vi "Write connect timeout ms.vi"(8 "error in (no error)":errorcluster, 10 "connect timeout ms":i32, 11 "TCP Master in":refnum<class "TCP Master.lvclass">) -> (0 "error out":errorcluster, 3 "TCP Master out":refnum<class "TCP Master.lvclass">)   [LabVIEW 2013, in "Modbus Library - Advance.lvlib" / "TCP Master.lvclass"]
uses:
  TCP Master.lvclass
  TCP Master.lvclass/TCP Master.ctl
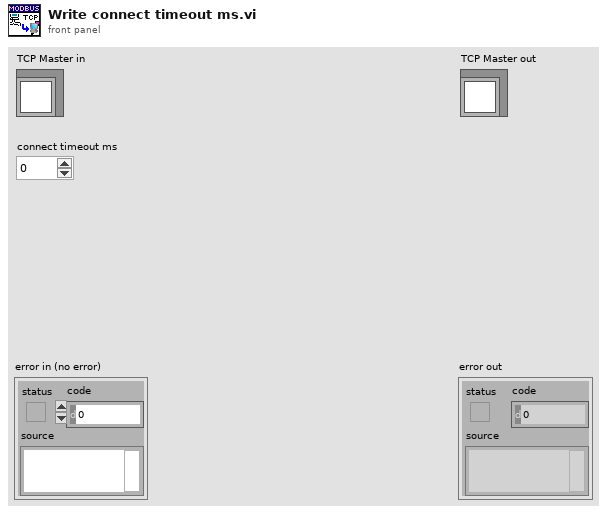
[diagram p1: front panel]
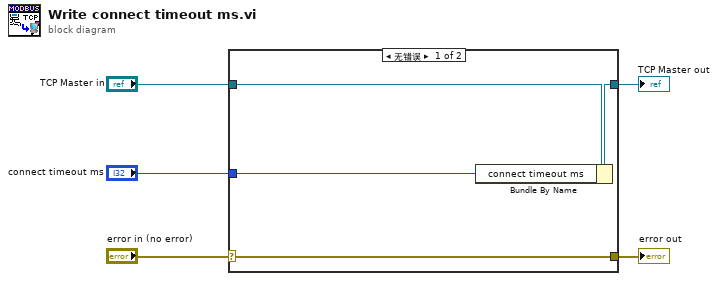
[diagram p0: block diagram]
diagram:
  n1 = case shown="无错误" "error in (no error)" {
    selector: "error in (no error)" -> [w9 w10]
    tunnel: [w9 w10] -> w4
    tunnel: [w7 w11] -> w2
    tunnel: "TCP Master in" -> [w8 w11]
    tunnel: "connect timeout ms" -> [w6 _]
    frame No Error {
      n2 = Bundle By Name(cluster=w8, "connect timeout ms"=w6) -> (w7:refnum<class "TCP Master.lvclass">)
    }
    frame Error {
    }
  }
  "error out" <- w4
  "TCP Master out" <- w2
